vi "CH_LM Config Trigger Source.vi"(0 "Meter Index":i32, 2 "Trigger Source":T1, 5 "error in (no error)":errorcluster, 7 "Timeout / ms (3000)":i32=3000, 8 "Action (query)":bool, 9 "Lock Timeout / ms (1000)":i32=1000) -> (11 "Lock timed out":bool, 14 "Meter Index":i32, 16 "Trigger Source":T1, 19 "error out":errorcluster)   [LabVIEW 2012, in "CH_LM.lvlib"]
doc: "This command will set/query the trigger source. (TOP Only)\n\n<B>Hint:</B> Selecting external trigger source will automatically result in internal trigger source selection when thermopile and optical probes are attached."
uses:
  CH_LM.lvlib
  CH_LM Trigger Source.ctl
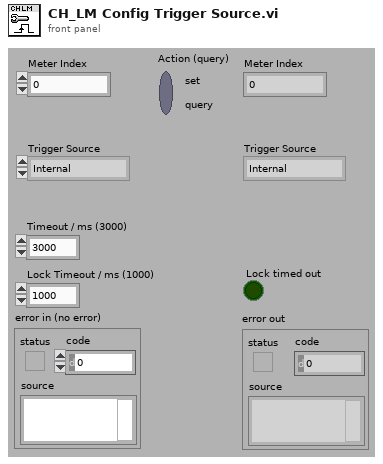
[diagram p1: front panel]
types:
  T1 = typedef "CH_LM.lvlib/CH_LM Trigger Source.ctl" = enum16{"Internal", "External", "Bus"}
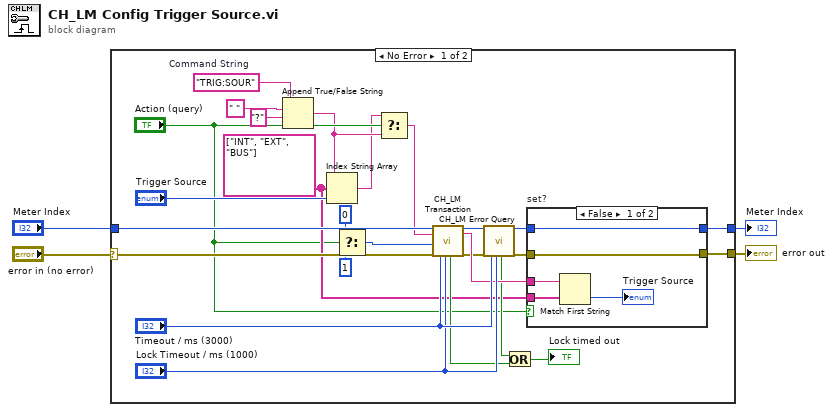
[diagram p0: block diagram]
diagram:
  n1 = case shown="No Error" "error in (no error)" {
    selector: "error in (no error)" -> [w30 w39]
    tunnel: [w28 w39] -> w4
    tunnel: "Meter Index" -> [w29 w38]
    tunnel: [w27 w38] -> w1
    frame No Error {
      w9 = string[] ["INT", "EXT", "BUS"] ("string array")
      w24 = "TRIG:SOUR"  # Command String
      n2 = Append True/False String(1:"Action (query)", 2:"?" ("true string"), 3:" ", 4:w24) -> (0:w7:string)
      n3 = Index String Array(1:"Trigger Source", 2:w9, 3:w7) -> (0:w6:string)
      n4 = Select(t=0, s="Action (query)", f=1 ("NofStrings (-1:all)")) -> (s? t:f=w20:i32)
      n5 = Select(t=w6, s="Action (query)", f=w7) -> (s? t:f=w5:string)
      n6 = call "CH_LM Transaction.vi"("Meter Index"=w29, "Command String"=w5, "NofStrings (-1:all)"=w20, "error in (no error)"=w30, "Timeout / ms (3000)"="Timeout / ms (3000)", "Lock Timeout / ms (1000)"="Lock Timeout / ms (1000)") -> ("Lock timed out"=w13:bool, "Meter Index"=w18:i32, "Response"=w23:string, "error out"=w16:errorcluster)  [unwired: 10 out]
      n7 = call "CH_LM Error Query.vi"("Meter Index"=w18, "error in (no error)"=w16, "Timeout / ms (3000)"="Timeout / ms (3000)", "Lock Timeout / ms (1000)"="Lock Timeout / ms (1000)") -> ("Lock timed out"=w14:bool, "Meter Index"=w17:i32, "error out"=w15:errorcluster)  [unwired: 13 out]
      n8 = Or(x=w14, y=w13) -> (x .or. y?=→"Lock timed out":bool)
      n9 = case "set?" shown="False" "Action (query)" {
        tunnel: w23 -> [w34 _]
        tunnel: w15 -> [w33 w37]
        tunnel: [w33 w37] -> w28
        tunnel: w17 -> [w35 w36]
        tunnel: [w35 w36] -> w27
        tunnel: w9 -> [w31 _]
        frame False {
          n10 = Match First String(2:w31, 3:w34) -> (0:→"Trigger Source":i32)  [unwired: 1 out]
        }
        frame True {
        }
      }
    }
    frame Error {
    }
  }
  "error out" <- w4
  "Meter Index" <- w1
